vi "Send Find Functions on Disk Message.vi"(8 "error in (no error)":errorcluster, 10 "Function Locations":path[](array[path]), 11 "Message Enqueuer in":refnum<class "Message Enqueuer.lvclass">) -> (0 "error out":errorcluster, 3 "Message Enqueuer out":refnum<class "Message Enqueuer.lvclass">)   [LabVIEW 2016, in "Controller Actor.lvlib" / "Find Functions On Disk Message.lvclass"]
uses:
  <userlib>/Common Components/Controller/Messages/Load Functions/Find Functions On Disk Message.lvclass
  <vilib>/ActorFramework/Message Enqueuer/Message Enqueuer.lvclass
  C:/Program Files (x86)/National Instruments/LabVIEW 2016/vi.lib/ActorFramework/Message/Message.lvclass
  <vilib>/ActorFramework/Message Enqueuer/Message Enqueuer.lvclass/Message Enqueuer.ctl
  <vilib>/ActorFramework/Message Priority Queue/Priority Enqueue.vi
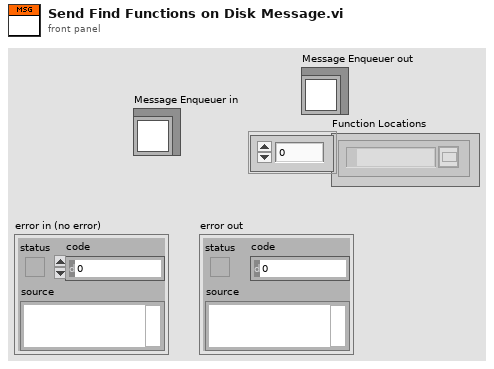
[diagram p1: front panel]
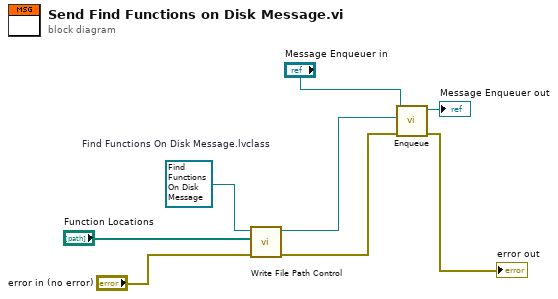
[diagram p0: block diagram]
diagram:
  w8 = refnum<class "Find Functions On Disk Message.lvclass"> refnum  # Find Functions On Disk Message.lvclass
  n1 = call <userlib>:"Write File Path Control.vi"("error in (no error)"="error in (no error)", "Function Locations"="Function Locations", "Load Functions Message in"=w8) -> ("error out"=w5:errorcluster, "Load Functions Message out"=w6:refnum<class "Find Functions On Disk Message.lvclass">)  [unwired: 7 in]
  n2 = call <vilib>:"Enqueue.vi"("error in (no error)"=w5, "Message"=w6, "Message Enqueuer in"="Message Enqueuer in") -> ("error out"=→"error out":errorcluster, "Message Enqueuer out"=→"Message Enqueuer out":refnum<class "Message Enqueuer.lvclass">)  [unwired: 7 in]
